vi "FestoCPX.Station.ProdSuctionGripper.Group.vi"(8 "error in":errorcluster, 10 "States in":bool[](array[boolean])) -> (0 "error out":errorcluster, 2 "States out":bool[](array[boolean]))   [LabVIEW 2016]
uses:
  FestoCPX.DO.Signal.ctl
  Station/Station.Global.vi
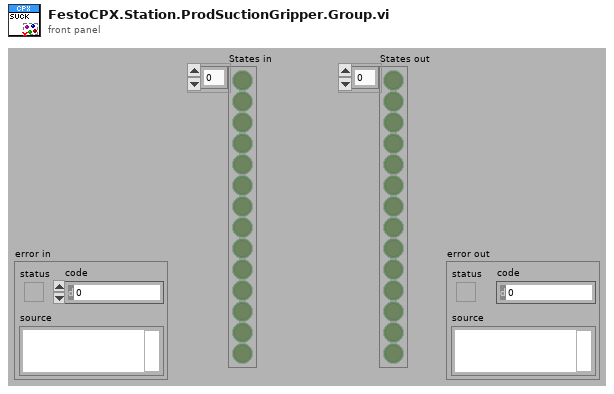
[diagram p1: front panel]
types:
  T1 = typedef "FestoCPX.DO.Signal.ctl" = enum16{"Safety Reset", "Air Main Valve", "Door Lock", "Button LED Start", "Button LED Stop", "Button LED Control", "Traffic LED Red", "Traffic LED Orange", "Traffic LED Green", "Horn", "Laser Interlock", "Laser Trigger", "Laser Fume Extractor", "Product Suction Gripper Slot 1 A", "Product Suction Gripper Slot 1 B", "Product Suction Gripper Slot 2 A", "Product Suction Gripper Slot 2 B", "Product Suction Gripper Slot 3 A", "Product Suction Gripper Slot 3 B", "Product Suction Gripper Slot 4 A", "Product Suction Gripper Slot 4 B", "Product Suction Gripper Final A", "Product Suction Gripper Final B", "Lamp", "Q1 Product Move Work", "Q1 Product Move Home", "Q2 Table Turn Work", "Q2 Table Turn Home", "Q3 Product Lift A", "Q3 Product Lift B", "Q4 Product Arm OK", "Q4 Product Arm NOK", "Q5 Product Arm Work", "Q6 Product BlowOut A", "Q6 Product BlowOut B"}
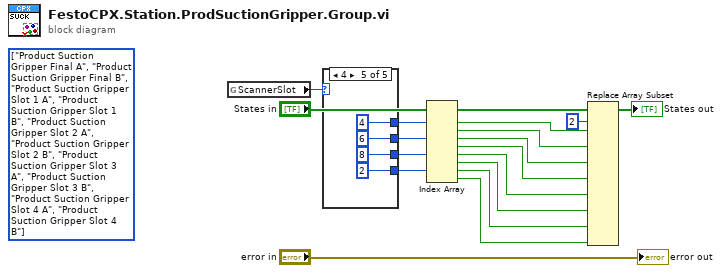
[diagram p0: block diagram]
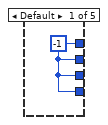
[diagram p2: hidden frame]
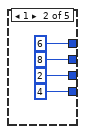
[diagram p3: hidden frame]
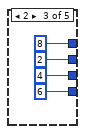
[diagram p4: hidden frame]
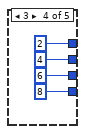
[diagram p5: hidden frame]
diagram:
  (unwired) T1[] [enum."Product Suction Gripper Final A", enum."Product Suction Gripper Final B", enum."Product Suction Gripper Slot 1 A", enum."Product Suction Gripper Slot 1 B", enum."Product Suction Gripper Slot 2 A", enum."Product Suction Gripper Slot 2 B", enum."Product Suction Gripper Slot 3 A", enum."Product Suction Gripper Slot 3 B", enum."Product Suction Gripper Slot 4 A", enum."Product Suction Gripper Slot 4 B"] items=["Safety Reset", "Air Main Valve", "Door Lock", "Button LED Start", "Button LED Stop", "Button LED Control", "Traffic LED Red", "Traffic LED Orange", "Traffic LED Green", "Horn", "Laser Interlock", "Laser Trigger", "Laser Fume Extractor", "Product Suction Gripper Slot 1 A", "Product Suction Gripper Slot 1 B", "Product Suction Gripper Slot 2 A", "Product Suction Gripper Slot 2 B", "Product Suction Gripper Slot 3 A", "Product Suction Gripper Slot 3 B", "Product Suction Gripper Slot 4 A", "Product Suction Gripper Slot 4 B", "Product Suction Gripper Final A", "Product Suction Gripper Final B", "Lamp", "Q1 Product Move Work", "Q1 Product Move Home", "Q2 Table Turn Work", "Q2 Table Turn Home", "Q3 Product Lift A", "Q3 Product Lift B", "Q4 Product Arm OK", "Q4 Product Arm NOK", "Q5 Product Arm Work", "Q6 Product BlowOut A", "Q6 Product BlowOut B"] ("CPX.DO")
  n1 = global read "Station.Global.vi" "ScannerSlot"() -> (w1:i32)
  n2 = case shown="4" w1 {
    tunnel: [w18 6 ("index") 8 ("index") 2 ("index") 4 ("index")] -> w14
    tunnel: [w18 8 ("index") 2 ("index") 4 ("index") 6 ("index")] -> w4
    tunnel: [w18 2 ("index") 4 ("index") 6 ("index") 8 ("index")] -> w3
    tunnel: [w18 4 ("index") 6 ("index") 8 ("index") 2 ("index")] -> w2
    frame Default {
      w18 = -1 ("index")
    }
    frame 1 {
    }
    frame 2 {
    }
    frame 3 {
    }
    frame 4 {
    }
  }
  n3 = Index Array(array="States in", index #1=w14, index #3=w4, index #5=w3, index #7=w2) -> (element #1=w13:bool, element #2=w11:bool, element #3=w10:bool, element #4=w9:bool, element #5=w8:bool, element #6=w7:bool, element #7=w6:bool, element #8=w5:bool)  [unwired: 4 in]
  n4 = Replace Array Subset(array="States in", new element #1=w13, index #1=2 ("index"), new element #2=w11, new element #3=w10, new element #4=w9, new element #5=w8, new element #6=w7, new element #7=w6, new element #8=w5) -> (→"States out":bool[])  [unwired: 7 in]
  "error out" <- "error in"
